vi "Run to State.vi"(8 "error in (no error)":errorcluster, 11 "BaseProducer in":refnum<class "BaseProducer.lvclass">) -> (0 "error out":errorcluster, 1 "Temperature Array (C)":dbl[](array[numeric]), 2 "Next State":string, 3 "BaseProducer out":refnum<class "BaseProducer.lvclass">)   [LabVIEW 2013, in "BaseProducer.lvclass"]
doc: "This method commands the system to move in a line from the current operating point to the desired operating point, stopping at steps along the way. For each step in Target Steps, this method commands the MFCs to follow a line from the current state to that step, then pauses at that step for one second to settle, and then one second of data collection. While moving, we only look for flame out. Once at the next step, we record data from all sensors. If flame out occurs, we skip to reignite, otherwise we go to next state."
uses:
  BaseProducer.lvclass
  BaseProducer.lvclass/BaseProducer.ctl
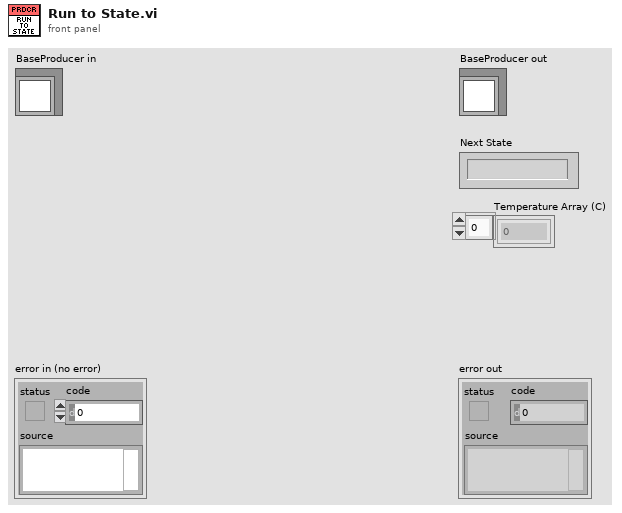
[diagram p1: front panel]
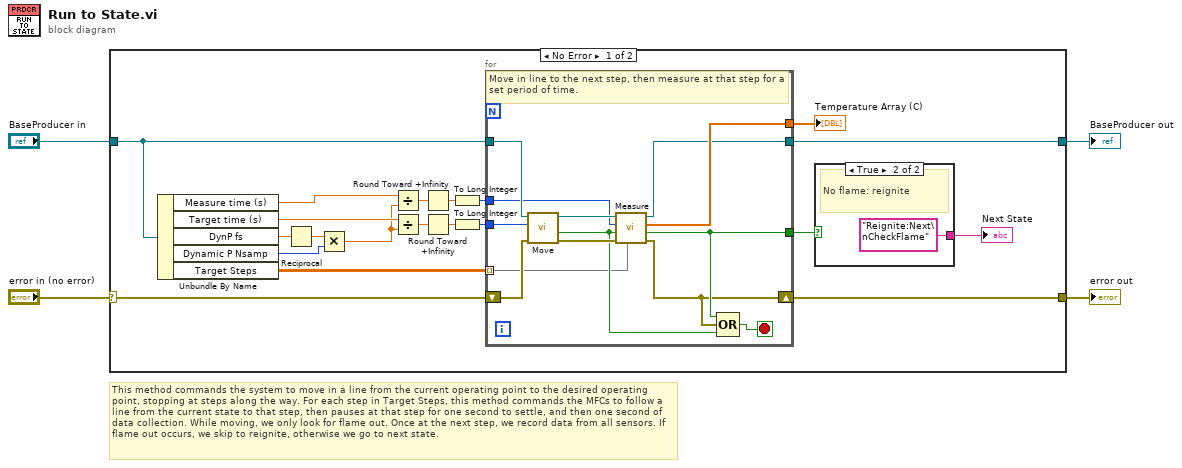
[diagram p0: block diagram]
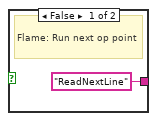
[diagram p2: hidden frame]
diagram:
  # "This method commands the system to move in a line from the current operating point to the desired operating point, stopping at steps along the way. For each step in Target Steps, this method commands the MFCs to follow a line from the current state to that step, then pauses at that step for one second to settle, and then one second of data collection. While moving, we only look for flame out. Once at the next step, we record data from all sensors. If flame out occurs, we skip to reignite, otherwise we go to next state."
  n1 = case shown="No Error" "error in (no error)" {
    selector: "error in (no error)" -> [w17 w41]
    tunnel: [w12 w41] -> w3
    tunnel: [w5 w40] -> w1
    tunnel: "BaseProducer in" -> [w16 w40]
    frame No Error {
      n2 = Unbundle By Name(w16) -> ("Measure time (s)"=w11:dbl, "Target time (s)"=w20:dbl, "DynP fs"=w22:dbl, "Dynamic P Nsamp"=w21:i32, "Target Steps"=w14:dbl[][])
      n3 = Reciprocal(x=w22) -> (1/x=w23:dbl)
      n4 = Multiply(x=w23, y=w21) -> (x*y=w10:dbl)
      n5 = Divide(x=w11, y=w10) -> (x/y=w9:dbl)
      n6 = Divide(x=w20, y=w10) -> (x/y=w19:dbl)
      n7 = Round Toward +Infinity(x=w9) -> (ceil(x): smallest int >= x=w8:dbl)
      n8 = Round Toward +Infinity(x=w19) -> (ceil(x): smallest int >= x=w18:dbl)
      n9 = To Long Integer(number=w8) -> (32bit integer=w7:i32)
      n10 = To Long Integer(number=w18) -> (32bit integer=w15:i32)
      n11 = for {
        tunnel: w16 -> [w29]
        tunnel: w15 -> [w36]
        shift-right: [w26] -> w12
        shift-left: w17 -> [w37]
        tunnel: w14 -> [w30] mode=indexing
        tunnel: [w33] -> w13
        tunnel: w7 -> [w28]
        tunnel: [w27] -> w6
        tunnel: [w25] -> w5
        stop <- w31 stop-if-true
        # "Move in line to the next step, then measure at that step for a set period of time."
        n12 = call "Move.vi"("error in (no error)"=w37, "Num Iterations"=w36, "BaseProducer in"=w29) -> ("error out"=w34:errorcluster, "Blow Out?"=w32:bool, "BaseProducer out"=w35:refnum<class "BaseProducer.lvclass">)  [unwired: 5 in, 1 out]
        n13 = call "Measure.vi"("Next Step"=w30, "error in (no error)"=w34, "Blow Out?"=w32, "Num Iterations"=w28, "BaseProducer in"=w35) -> ("error out"=w26:errorcluster, "Blow Out?"=w33:bool, "Temperature Array (C)"=w27:dbl[], "BaseProducer out"=w25:refnum<class "BaseProducer.lvclass">)  [unwired: 3 in]
        n14 = Compound Arithmetic op=OR(w33, w26, w32) -> (w31:bool)
      }
      "Temperature Array (C)" <- w6
      n15 = case shown="True" w13 {
        tunnel: ["ReadNextLine" "Reignite:Next\nCheckFlame"] -> w24
        frame False {
          # "Flame: Run next op point"
        }
        frame True {
          # "No flame: reignite"
        }
      }
      "Next State" <- w24
    }
    frame Error {
    }
  }
  "error out" <- w3
  "BaseProducer out" <- w1
